vi "Parameters_Build_PositionMove.vi"(8 "Acceleration Jerk":dbl=1000.0, 9 "Acceleration":dbl=10000.0, 10 "Velocity":dbl=1000.0, 11 "Positions":dbl[](array[numeric])) -> (3 "Parameters":dbl[](array[numeric]))   [LabVIEW 2017, in "WordManipulationLibrary.lvlib"]
uses:
  WordManipulationLibrary.lvlib
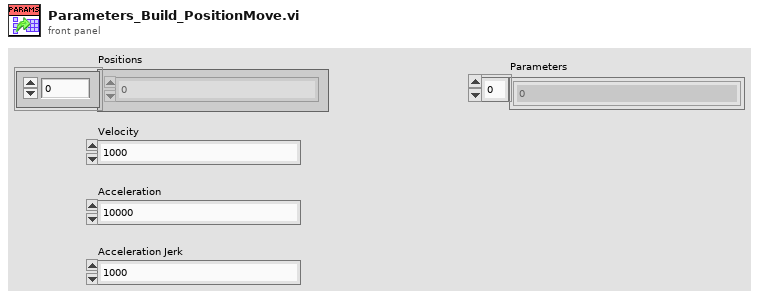
[diagram p1: front panel]
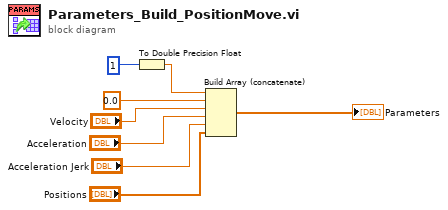
[diagram p0: block diagram]
diagram:
  n1 = To Double Precision Float(number=i16 1 ("element")) -> (double precision float=w1:dbl)
  n2 = Build Array (concatenate)(w1, 0.0 ("element"), "Velocity", "Acceleration", "Acceleration Jerk", "Positions") -> (→"Parameters":dbl[])
